vi "niFpgaFFTStreamingStages_4096.vi"(0 "reset":bool, 1 "mult output type":fxp<+/-,18,2> format="%#.17g", 2 "bf bullet type":fxp<+,7,7>, 5 "bf data in":T1 {"x_r" format="%.16g"; "x_i" format="%.16g"; "y_r" format="%.16g"; "y_i" format="%.16g"}, 7 "stage switch in":bool, 9 "twiddle index in":fxp<+,6,6>, 11 "bf data type":T1 {"x_r" format="%.16g"; "x_i" format="%.16g"; "y_r" format="%.16g"; "y_i" format="%.16g"}) -> (6 "bf data out":T1 {"x_r" format="%.16g"; "x_i" format="%.16g"; "y_r" format="%.16g"; "y_i" format="%.16g"}, 8 "stage switch out":bool)   [LabVIEW 2017]
uses:
  <vilib>/rvi/Analysis/measure/FFT/supportingXNodes/permutation/templates/niFPGA FFT Perm Buffer 1024 U32.vi
  <vilib>/rvi/Analysis/measure/FFT/supportingXNodes/BFGroup/templates/niFPGA BFGroup Input Buffer 4096 U32.vi
  <vilib>/rvi/Analysis/measure/FFT/supportingXNodes/BFGroup/templates/niFPGA BFGroup Twiddle Table 2048 U32.vi
  <vilib>/rvi/Analysis/measure/FFT/supportingXNodes/permutation/templates/niFPGA FFT Perm Buffer 256 U32.vi
  <vilib>/rvi/Analysis/measure/FFT/supportingXNodes/permutation/templates/niFPGA FFT Perm Buffer 512 U32.vi
  <vilib>/rvi/Analysis/measure/FFT/supportingXNodes/BFGroup/templates/niFPGA BFGroup Twiddle Table 512 U32.vi
  <vilib>/rvi/Analysis/measure/FFT/supportingXNodes/permutation/templates/niFPGA FFT Perm Buffer 64 U32.vi
  <vilib>/rvi/Analysis/measure/FFT/supportingXNodes/permutation/templates/niFPGA FFT Perm Buffer 128 U32.vi
  <vilib>/rvi/Analysis/measure/FFT/supportingXNodes/BFGroup/templates/niFPGA BFGroup Twiddle Table 128 U32.vi
  <vilib>/rvi/Analysis/measure/FFT/supportingXNodes/BFGroup/templates/niFPGA BFGroup Twiddle Table 32 U32.vi
  <vilib>/rvi/Analysis/measure/FFT/supportingXNodes/BFGroup/templates/niFPGA BFGroup Twiddle Table 8 U32.vi
  <vilib>/rvi/Analysis/measure/FFT/supportingXNodes/BFGroup/XNode/niFpgaFFTBFGroup.xnode
  <vilib>/rvi/FXPMathLib/basic elements/FxpDiscreteDelay/XNode/nifxpmath_DiscreteDelay.xnode
  <vilib>/rvi/Analysis/measure/FFT/supportingXNodes/permutation/XNode/niFpgaFFTPermutation.xnode
  <vilib>/rvi/Analysis/measure/FFT/supportingXNodes/butterfly/XNode/niFpgaFFTDIFButterfly.xnode
  <vilib>/rvi/FXPMathLib/FxpMul/XNode/nifxpmath_Multiplier.xnode
  <vilib>/rvi/FXPMathLib/sim/FxpSim.dll
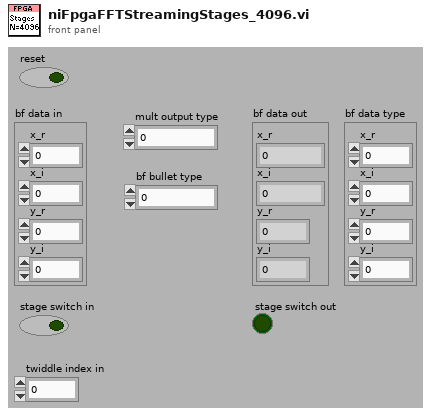
[diagram p1: front panel]
types:
  T1 = cluster{"x_r":fxp<+/-,16,1>, "x_i ":fxp<+/-,16,1>, "y_r ":fxp<+/-,16,1>, "y_i ":fxp<+/-,16,1>}
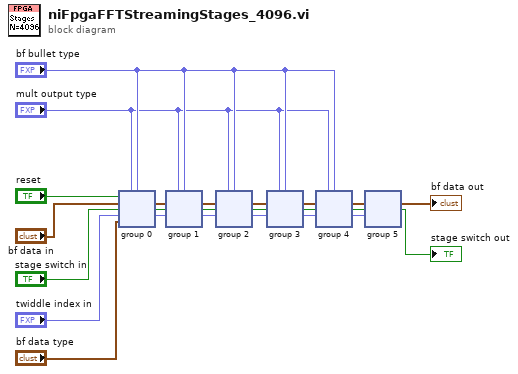
[diagram p0: block diagram]
diagram:
  n1 = xnode "group 0"("mult output type"="mult output type", "bf data in"="bf data in", "stage switch in"="stage switch in", "tf index in"="twiddle index in", "reset"="reset", "bf bullet type"="bf bullet type", "bf data type"="bf data type") -> ("stage switch out"=w24:bool, "bf data out"=w14:T1, "tf index out"=w23:fxp<+,11,11>)
  n2 = xnode "group 1"("mult output type"="mult output type", "bf data in"=w14, "stage switch in"=w24, "tf index in"=w23, "bf bullet type"="bf bullet type") -> ("stage switch out"=w22:bool, "bf data out"=w13:T1, "tf index out"=w21:fxp<+,11,11>)
  n3 = xnode "group 2"("mult output type"="mult output type", "bf data in"=w13, "stage switch in"=w22, "tf index in"=w21, "bf bullet type"="bf bullet type") -> ("stage switch out"=w20:bool, "bf data out"=w12:T1, "tf index out"=w19:fxp<+,11,11>)
  n4 = xnode "group 3"("mult output type"="mult output type", "bf data in"=w12, "stage switch in"=w20, "tf index in"=w19, "bf bullet type"="bf bullet type") -> ("stage switch out"=w18:bool, "bf data out"=w11:T1, "tf index out"=w17:fxp<+,11,11>)
  n5 = xnode "group 4"("mult output type"="mult output type", "bf data in"=w11, "stage switch in"=w18, "tf index in"=w17, "bf bullet type"="bf bullet type") -> ("stage switch out"=w15:bool, "bf data out"=w10:T1, "tf index out"=w16:fxp<+,11,11>)
  n6 = xnode "group 5"("bf data in"=w10, "stage switch in"=w15, "tf index in"=w16) -> ("stage switch out"=→"stage switch out":bool, "bf data out"=→"bf data out":T1)
